vi "StopFPGA.vi"(8 "error in":errorcluster, 11 "FPGASession in":refnum<class "FPGASession.lvclass">) -> (0 "error out":errorcluster, 3 "FPGASession out":refnum<class "FPGASession.lvclass">)   [LabVIEW 2013, in "FPGASession.lvclass"]
uses:
  FPGASession.lvclass
  FPGASession.lvclass/FPGASession.ctl
  <vilib>/FPGAPlugInAG/sbRIO-9636/niLvFpga_Close_sbRIO-9636.vi
  <vilib>/rvi/interface/nirviMethod/nirviMethod.xnode
  RT/FPGASession/FPGARef.ctl
  FPGA Bitfiles/HWSWTriggerBox_FPGATarget2_TriggerBox_1zhzIx5zPP8.lvbitx
  FPGAMain.vi
  <vilib>/rvi/interface/nirviCloseFPGA/nirviCloseFPGA.xnode
  <vilib>/FPGAPlugInAG/sbRIO-9636/niLvFpga_Abort_sbRIO-9636.vi
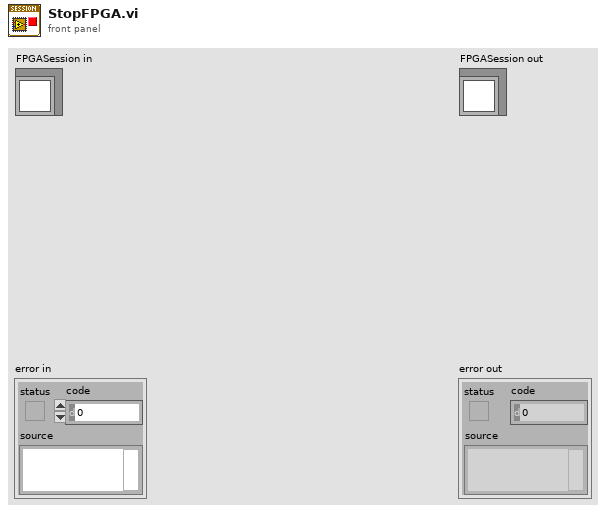
[diagram p1: front panel]
types:
  T1 = typedef "FPGASession.lvclass/FPGARef.ctl" = refnum<k20>
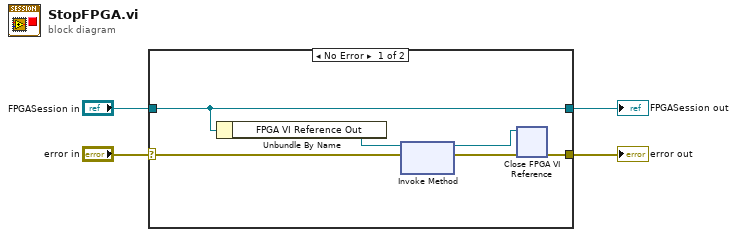
[diagram p0: block diagram]
diagram:
  n1 = case shown="No Error" "error in" {
    selector: "error in" -> [w8 w12]
    tunnel: [w5 w12] -> w3
    tunnel: [w10 w11] -> w1
    tunnel: "FPGASession in" -> [w10 w11]
    frame No Error {
      n2 = Unbundle By Name(w10) -> ("FPGA VI Reference Out"=w9:T1)
      n3 = xnode "Invoke Method"("FPGA VI Reference In"=w9, "error in"=w8) -> ("FPGA VI Reference Out"=w7:T1, "error out"=w6:errorcluster)
      n4 = xnode "Close FPGA VI Reference"("FPGA VI Reference In"=w7, "error in"=w6) -> ("error out"=w5:errorcluster)
    }
    frame Error {
    }
  }
  "error out" <- w3
  "FPGASession out" <- w1
